vi "Velocity&AccelerationCalc.vi"(2 "Pulses/Revolution":dbl, 3 "Fixed Time \nInterval (uSec)":dbl, 4 "Acceleration (Counts/Interval)":i32, 5 "Velocity (Counts/Interval)":i32) -> (0 "Acceleration (rps/s)":dbl, 1 "Velocity (RPM)":dbl)   [LabVIEW 2015]
doc: "This vi takes as inputs the velocity and acceleration of a quadrature encoder in counts/interval, received from the Encoder Position & Velocity (FPGA).vi and computes velocity in rpm and acceleration in rps/s. The vi also requires as inputs counts/revolution of the quadrature encoder and the fixed time interval used for velocity and acceleration estimation."
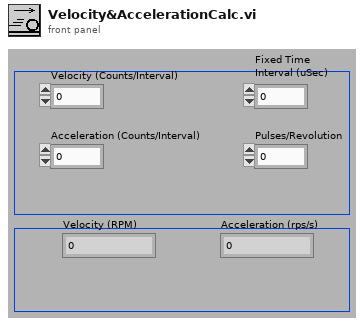
[diagram p1: front panel]
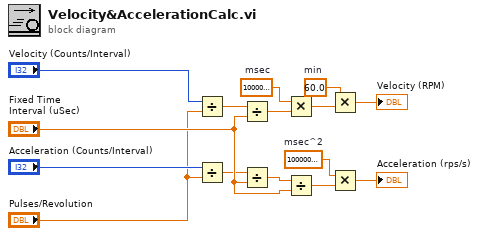
[diagram p0: block diagram]
diagram:
  w14 = 1000000000000.0  # msec^2
  w8 = 60.0  # min
  w5 = 1000000.0  # msec
  n1 = Divide(x="Velocity (Counts/Interval)", y="Pulses/Revolution") -> (x/y=w3:dbl)
  n2 = Divide(x="Acceleration (Counts/Interval)", y="Pulses/Revolution") -> (x/y=w1:dbl)
  n3 = Divide(x=w3, y="Fixed Time \nInterval (uSec)") -> (x/y=w4:dbl)
  n4 = Divide(x=w1, y="Fixed Time \nInterval (uSec)") -> (x/y=w11:dbl)
  n5 = Multiply(x=w5, y=w4) -> (x*y=w7:dbl)
  n6 = Divide(x=w11, y="Fixed Time \nInterval (uSec)") -> (x/y=w13:dbl)
  n7 = Multiply(x=w8, y=w7) -> (x*y=→"Velocity (RPM)":dbl)
  n8 = Multiply(x=w14, y=w13) -> (x*y=→"Acceleration (rps/s)":dbl)
